vi "报警弹出信息.vi"(10 "Diaplay Info":string) -> (2 "OK?":bool)   [LabVIEW 2018]
panel:
  out "Display Info":string
  in  "Ok":bool
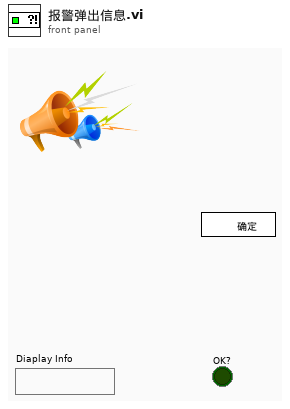
[diagram p1: front panel]
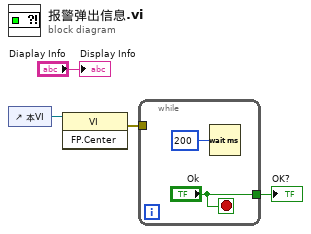
[diagram p0: block diagram]
diagram:
  n1 = control-ref of="本VI"() -> (w2:refnum<vi>)
  n2 = invoke class="VI" method="FP.Center"(reference=w2) -> (error out=w1:errorcluster)  [unwired: 2 in, 2 out]
  n3 = while {
    tunnel: ["Ok"] -> w3
    tunnel: w1 -> [_]
    stop <- "Ok" stop-if-true
    n4 = Wait (ms)(milliseconds to wait=u32 200 ("等待时间（毫秒）")) -> ()  [unwired: 1 out]
  }
  "OK?" <- w3
  "Display Info" <- "Diaplay Info"
